vi "CalcDivideDigits.vi"(1 "Digits":i32, 2 "decimal Ofst":i32, 3 "Array Size":i32) -> (0 "decimal Ofst 2":i32)   [LabVIEW 2025]
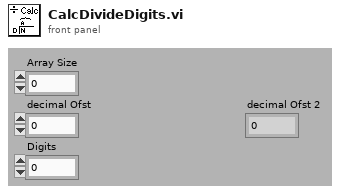
[diagram p1: front panel]
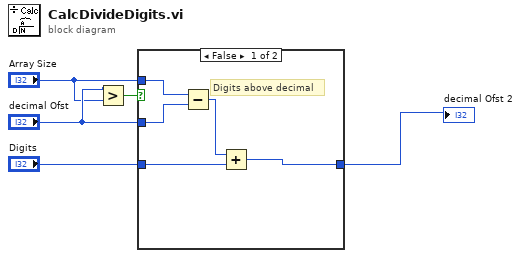
[diagram p0: block diagram]
diagram:
  n1 = Greater?(x="decimal Ofst", y="Array Size") -> (0:w5:bool)
  n2 = case shown="False" w5 {
    tunnel: "Digits" -> [w7 w11]
    tunnel: "decimal Ofst" -> [w9 _]
    tunnel: "Array Size" -> [w10 _]
    tunnel: [w6 w11] -> w1
    frame False {
      # "Digits above decimal"
      n3 = Subtract(x=w10, y=w9) -> (x-y=w8:i32)
      n4 = Add(x=w8, y=w7) -> (x+y=w6:i32)
    }
    frame True {
    }
  }
  "decimal Ofst 2" <- w1
